vi "Pass active channel values to memory.vi"(8 "Module":i32, 10 "Active channels":T1(array[cluster])=[{"Active channels"=[], "Memory offset"=0}, {"Active channels"=[], "Memory offset"=0}, {"Active channels"=[], "Memory offset"=0}, {"Active channels"=[], "Memory offset"=0}, {"Active channels"=[], "Memory offset"=0}, {"Active channels"=[], "Memory offset"=0}, {"Active channels"=[], "Memory offset"=0}, {"Active channels"=[], "Memory offset"=0}], 11 "Acquired data":sgl[](array[numeric])=[0.0, 0.0, 0.0, 0.0, 0.0, 0.0, 0.0, 0.0, 0.0, 0.0, 0.0, 0.0, 0.0, 0.0, 0.0, 0.0, 0.0, 0.0, 0.0, 0.0, 0.0, 0.0, 0.0, 0.0, 0.0, 0.0, 0.0, 0.0, 0.0, 0.0, 0.0, 0.0]) -> ()   [LabVIEW 2018]
uses:
  <vilib>/rvi/Memory/Memory_Emulation/nirvimemoryFastEmulation.vi
  <vilib>/rvi/Memory/Memory_Emulation/nirvimemoryEmulation.vi
  <vilib>/rvi/Emulation/niFpgaEmulationIsFPGAContextNoSignature.vi
  <vilib>/rvi/DataTransferAndStorage/Container/Common/niFpgaContainerGetUniqueNameForEmu.vi
  <vilib>/rvi/Emulation/niFpgaProcessEmulError.vi
  <vilib>/rvi/Emulation/niFpgaSctlEmulationGetInTimedLoop.vi
  <vilib>/rvi/errors/nirviReportUnexpectedCaseInternalError (U32).vi
  <vilib>/rvi/DataTransferAndStorage/Container/XNode/niFpgaContainer.xnode
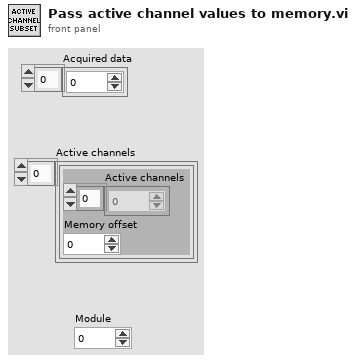
[diagram p1: front panel]
types:
  T1 = cluster{"Active channels":u8[], "Memory offset":i16}[]
  T2 = cluster{"Active channels":u8[], "Memory offset":i16}
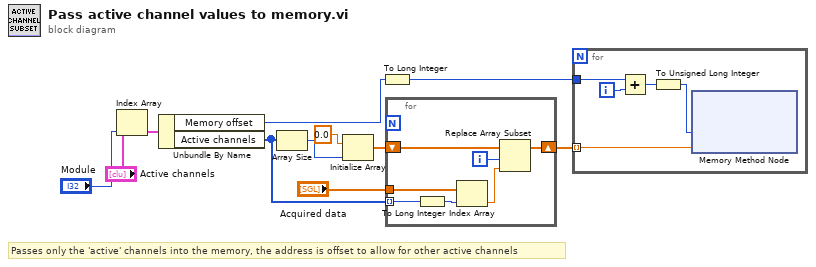
[diagram p0: block diagram]
diagram:
  # "Passes only the 'active' channels into the memory, the address is offset to allow for other active channels"
  n1 = Index Array(array="Active channels", index="Module") -> (element=w11:T2)
  n2 = Unbundle By Name(w11) -> ("Memory offset"=w2:i16, "Active channels"=w6:u8[])
  n3 = Array Size(array=w6) -> (size(s)=w9:i32)
  n4 = Initialize Array(sgl 0.0, w9) -> (w7:sgl[])
  n5 = To Long Integer(number=w2) -> (32bit integer=w1:i32)
  n6 = for {
    tunnel: "Acquired data" -> [w18]
    shift-right: [w14] -> w5
    shift-left: w7 -> [w17]
    tunnel: w6 -> [w13] mode=indexing
    i -> [w15]
    n7 = To Long Integer(number=w13) -> (32bit integer=w12:i32)
    n8 = Index Array(array=w18, index=w12) -> (element=w16:sgl)
    n9 = Replace Array Subset(array=w17, new element=w16, index=w15) -> (w14:sgl[])
  }
  n10 = for {
    tunnel: w5 -> [w22] mode=indexing
    tunnel: w1 -> [w20]
    i -> [w23]
    n11 = Add(x=w20, y=w23) -> (x+y=w21:i32)
    n12 = To Unsigned Long Integer(number=w21) -> (unsigned 32bit integer=w19:u32)
    n13 = xnode ("Memory Method Node")("Address"=w19, "Data"=w22) -> ()  [unwired: 1 in, 1 out]
  }
